vi "Food_Ordering.vi"() -> ()   [LabVIEW 2019]
panel:
  in  "?":bool
  in  "?":bool
  in  "?":enum32{"Page 1", "Page 2"}(tab)
  in  "?":bool
  out "TOTAL":dbl
  in  "PAROTTA":bool
  in  "Quantity  4":dbl=10.0 min=1.0 max=10.0 step=1.0
  out "Price   3":dbl
  in  "CHAPPATHI":bool
  in  "Quantity  3":dbl=10.0 min=1.0 max=10.0 step=1.0
  out "Price   2":dbl
  in  "VARIETY RICE":bool
  in  "Quantity  2":dbl=10.0 min=1.0 max=10.0 step=1.0
  out "Price":dbl
  in  "VEG MEALS":bool
  in  "Quantity":dbl=10.0 min=1.0 max=10.0 step=1.0
  out "Price":dbl
  out "Price":dbl
  in  "Quantity":dbl=10.0 min=1.0 max=10.0 step=1.0
  in  "NON VEG MEALS":bool
  in  "CHICKEN BRIYANI":bool
  in  "Quantity":dbl=10.0 min=1.0 max=10.0 step=1.0
  out "Price":dbl
  in  "MUTTON BRIYANI":bool
  in  "Quantity":dbl=10.0 min=1.0 max=10.0 step=1.0
  out "Price":dbl
  in  "PRAWN BRIYANI":bool
  in  "Quantity":dbl=10.0 min=1.0 max=10.0 step=1.0
  out "Price":dbl
  out "TOTAL":dbl
  in  "?":bool
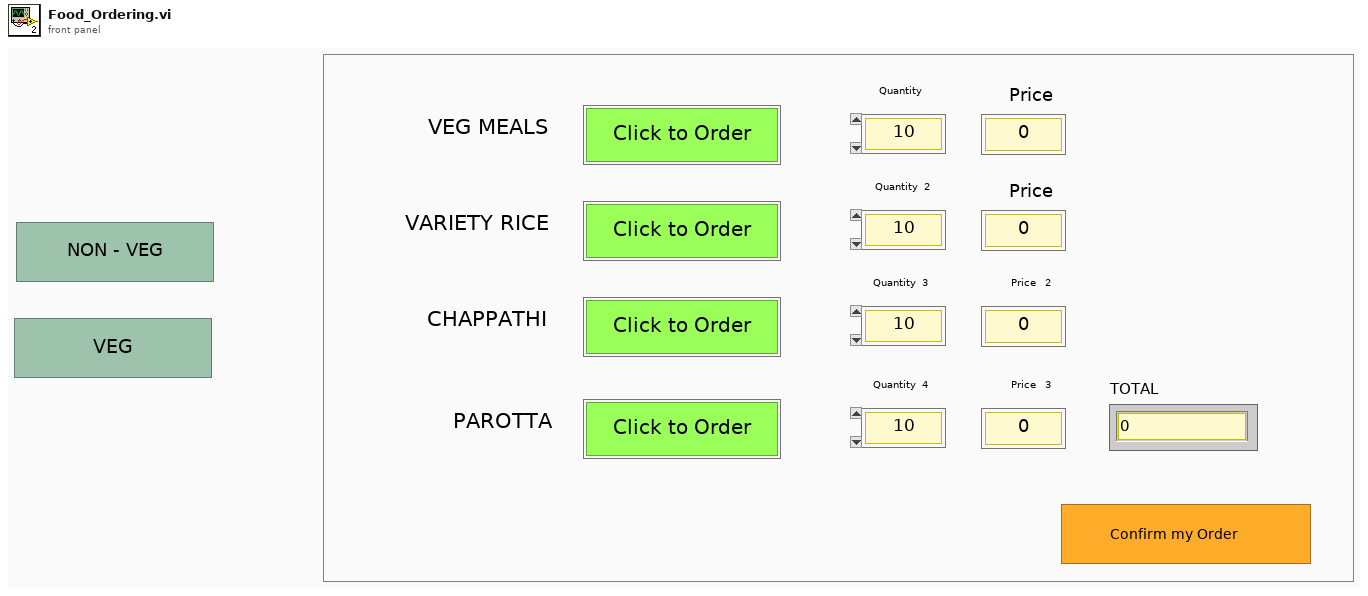
[diagram p1: front panel]
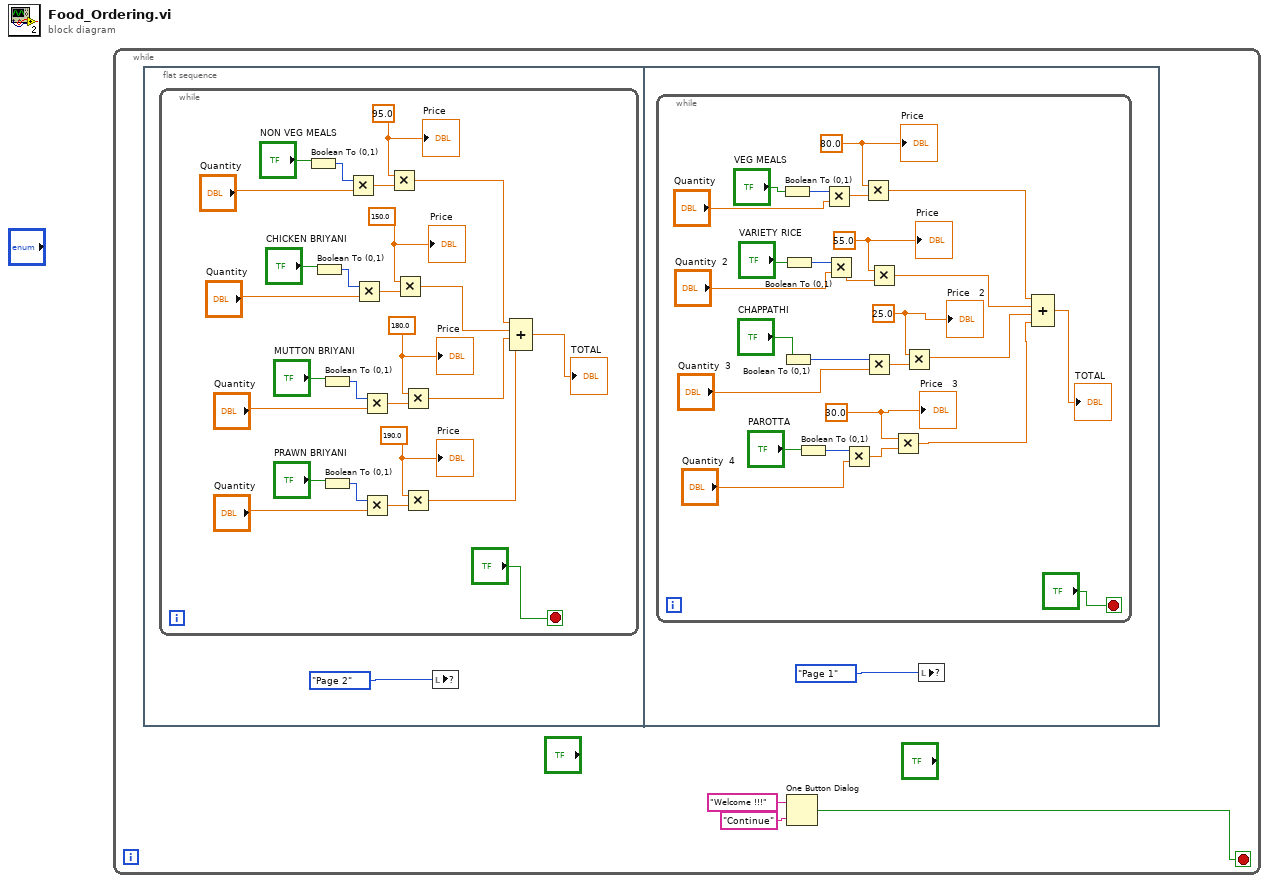
[diagram p0: block diagram]
diagram:
  n1 = while {
    stop <- w3 stop-if-true
    n2 = flat-sequence {
      frame #0 {
        n3 = while {
          stop <- "?" stop-if-true
          w11 = 190.0 ("Price")
          w16 = 180.0 ("Price")
          w21 = 150.0 ("Price")
          w26 = 95.0 ("Price")
          n4 = Boolean To (0,1)(Boolean="NON VEG MEALS") -> (0, 1=w29:i16)
          n5 = Boolean To (0,1)(Boolean="CHICKEN BRIYANI") -> (0, 1=w24:i16)
          n6 = Boolean To (0,1)(Boolean="MUTTON BRIYANI") -> (0, 1=w19:i16)
          n7 = Boolean To (0,1)(Boolean="PRAWN BRIYANI") -> (0, 1=w14:i16)
          n8 = Multiply(x=w29, y="Quantity") -> (x*y=w27:dbl)
          n9 = Multiply(x=w24, y="Quantity") -> (x*y=w22:dbl)
          n10 = Multiply(x=w19, y="Quantity") -> (x*y=w17:dbl)
          n11 = Multiply(x=w14, y="Quantity") -> (x*y=w12:dbl)
          n12 = Multiply(x=w26, y=w27) -> (x*y=w9:dbl)
          n13 = Multiply(x=w21, y=w22) -> (x*y=w8:dbl)
          n14 = Multiply(x=w16, y=w17) -> (x*y=w7:dbl)
          n15 = Multiply(x=w11, y=w12) -> (x*y=w6:dbl)
          n16 = Compound Arithmetic op=ADD(w9, w8, w7, w6) -> (→"TOTAL":dbl)
          "Price" <- w26
          "Price" <- w21
          "Price" <- w16
          "Price" <- w11
        }
        n17 = local write item#?(enum32{"Page 1", "Page 2"}."Page 2" ("Tab Control")) -> ()
      }
      frame #1 {
        n18 = while {
          stop <- "?" stop-if-true
          w37 = 30.0 ("Price   3")
          w42 = 25.0 ("Price   2")
          w47 = 55.0 ("Price")
          w53 = 80.0 ("Price")
          n19 = Boolean To (0,1)(Boolean="VEG MEALS") -> (0, 1=w55:i16)
          n20 = Boolean To (0,1)(Boolean="CHAPPATHI") -> (0, 1=w45:i16)
          n21 = Boolean To (0,1)(Boolean="VARIETY RICE") -> (0, 1=w50:i16)
          n22 = Boolean To (0,1)(Boolean="PAROTTA") -> (0, 1=w40:i16)
          n23 = Multiply(x=w55, y="Quantity") -> (x*y=w57:dbl)
          n24 = Multiply(x=w50, y="Quantity  2") -> (x*y=w51:dbl)
          n25 = Multiply(x=w40, y="Quantity  4") -> (x*y=w38:dbl)
          n26 = Multiply(x=w53, y=w57) -> (x*y=w36:dbl)
          n27 = Multiply(x=w45, y="Quantity  3") -> (x*y=w43:dbl)
          n28 = Multiply(x=w47, y=w51) -> (x*y=w35:dbl)
          n29 = Multiply(x=w37, y=w38) -> (x*y=w33:dbl)
          n30 = Multiply(x=w42, y=w43) -> (x*y=w34:dbl)
          n31 = Compound Arithmetic op=ADD(w36, w35, w34, w33) -> (→"TOTAL":dbl)
          "Price" <- w53
          "Price" <- w47
          "Price   2" <- w42
          "Price   3" <- w37
        }
        n32 = local write item#?(enum32{"Page 1", "Page 2"}."Page 1" ("Tab Control")) -> ()
      }
    }
    n33 = One Button Dialog(message="Welcome !!!", button name ("OK")="Continue" ("F button name (\"Cancel\")")) -> (true=w3:bool)
  }
